vi "DSC TSV to PGSQL Record Processed.vi"() -> ()   [LabVIEW 2019]
panel:
  in  "path":path
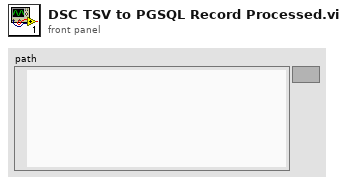
[diagram p1: front panel]
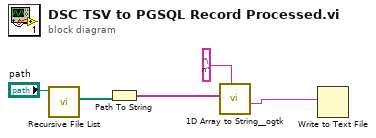
[diagram p0: block diagram]
diagram:
  n1 = call <vilib>:"Recursive File List.vi"("Folder Path"="path") -> ("All Files in Dir"=w2:path[])  [unwired: 6 in, 4 out]
  n2 = Path To String(path=w2) -> (string=w4:string[])
  n3 = call <userlib>:"1D Array to String__ogtk.vi"("delimiter (Tab)"="\n", "Array of Strings"=w4) -> ("delimited string"=w3:string)  [unwired: 9 in]
  n4 = Write to Text File(text=w3) -> ()  [unwired: 3 in, 3 out]
